vi "calculatewidth.vi"(8 "Ch2 Width/Duty":bool, 9 "Ch1 Width/Duty":bool, 11 "Pulse Gen Basic Scan.lvclass":refnum<class "Pulse Gen Basic Scan.lvclass">) -> (0 "Ch2 Width":dbl[unit], 1 "Ch1 Width":dbl[unit], 3 "Pulse Gen Basic Scan.lvclass 2":refnum<class "Pulse Gen Basic Scan.lvclass">, 4 "Ch2 %Duty":dbl, 6 "Ch1 %Duty":dbl)   [LabVIEW 2023, in "Pulse Gen Basic Scan.lvclass"]
uses:
  Pulse Gen Basic Scan.lvclass
  Pulse Gen Basic Scan.lvclass/Pulse Gen Basic Scan.ctl
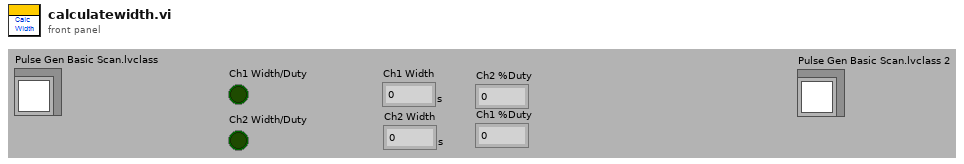
[diagram p1: front panel]
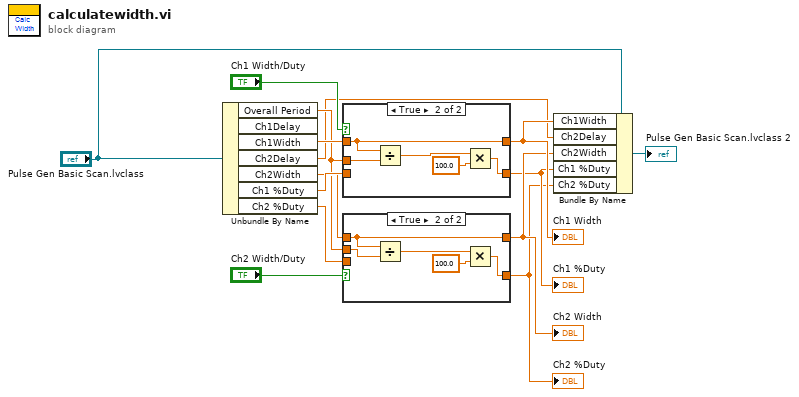
[diagram p0: block diagram]
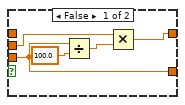
[diagram p2: hidden frame]
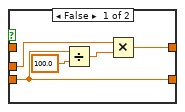
[diagram p3: hidden frame]
diagram:
  n1 = Unbundle By Name("Pulse Gen Basic Scan.lvclass") -> ("Overall Period"=w8:dbl[unit], "Ch1Width"=w13:dbl[unit], "Ch2Delay"=w3:dbl[unit], "Ch2Width"=w10:dbl[unit], "Ch1 %Duty"=w12:dbl, "Ch2 %Duty"=w9:dbl)  [unwired: 1 out]
  n2 = case shown="True" "Ch1 Width/Duty" {
    tunnel: w13 -> [_ w23]
    tunnel: [w16 w23] -> w5
    tunnel: w8 -> [w17 w24]
    tunnel: w12 -> [w15 _]
    tunnel: [w15 w20] -> w2
    frame False {
      n3 = Divide(x=w15, y=100.0) -> (x/y=w18:dbl)
      n4 = Multiply(x=w17, y=w18) -> (x*y=w16:dbl[unit])
    }
    frame True {
      n5 = Divide(x=w23, y=w24) -> (x/y=w22:dbl)
      n6 = Multiply(x=w22, y=100.0) -> (x*y=w20:dbl)
    }
  }
  "Ch1 Width" <- w5
  "Ch1 %Duty" <- w2
  n7 = case shown="True" "Ch2 Width/Duty" {
    tunnel: w10 -> [_ w33]
    tunnel: [w26 w33] -> w4
    tunnel: w9 -> [w25 _]
    tunnel: w8 -> [w27 w34]
    tunnel: [w25 w30] -> w1
    frame False {
      n8 = Divide(x=w25, y=100.0) -> (x/y=w28:dbl)
      n9 = Multiply(x=w27, y=w28) -> (x*y=w26:dbl[unit])
    }
    frame True {
      n10 = Divide(x=w33, y=w34) -> (x/y=w31:dbl)
      n11 = Multiply(x=w31, y=100.0) -> (x*y=w30:dbl)
    }
  }
  "Ch2 Width" <- w4
  "Ch2 %Duty" <- w1
  n12 = Bundle By Name(cluster="Pulse Gen Basic Scan.lvclass", "Ch1Width"=w5, "Ch2Delay"=w3, "Ch2Width"=w4, "Ch1 %Duty"=w2, "Ch2 %Duty"=w1) -> (→"Pulse Gen Basic Scan.lvclass 2":refnum<class "Pulse Gen Basic Scan.lvclass">)
